vi "Display.vi"(8 "error in (no error)":errorcluster, 11 "[V] User List in":refnum<class "[V] User List.lvclass">) -> (0 "error out":errorcluster, 3 "[V] User List out":refnum<class "[V] User List.lvclass">)   [LabVIEW 2020, in "[V] User List.lvlib" / "[V] User List.lvclass"]
uses:
  [V] User List.lvclass
  [V] User List.lvclass/[V] User List.ctl
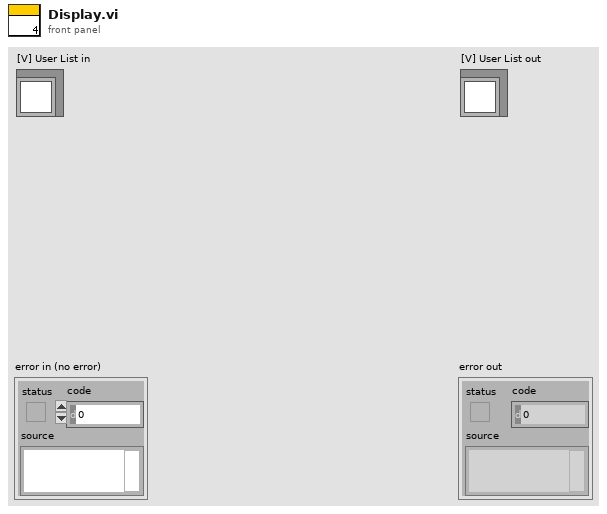
[diagram p1: front panel]
types:
  T1 = typedef "[V] User List.lvlib/[V] User List.lvclass/User Info List.ctl" = cluster{"username":string, "authority":string, "department":string, "post":string, "remark":string, "create time":timestamp, "last login time":timestamp}[]
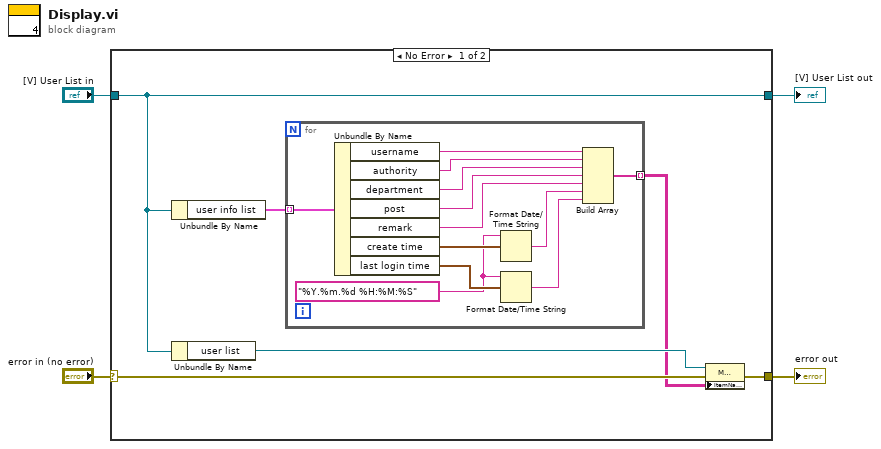
[diagram p0: block diagram]
diagram:
  n1 = case shown="No Error" "error in (no error)" {
    selector: "error in (no error)" -> [w8 w24]
    tunnel: [w5 w24] -> w3
    tunnel: [w9 w23] -> w1
    tunnel: "[V] User List in" -> [w9 w23]
    frame No Error {
      n2 = Unbundle By Name(w9) -> ("user info list"=w10:T1)
      n3 = Unbundle By Name(w9) -> ("user list"=w7:refnum<vi>)
      n4 = for {
        tunnel: w10 -> [w22] mode=indexing
        tunnel: [w16] -> w6 mode=indexing
        w11 = "%Y.%m.%d %H:%M:%S" ("time format string (%c)")
        n5 = Unbundle By Name(w22) -> ("username"=w21:string, "authority"=w17:string, "department"=w20:string, "post"=w19:string, "remark"=w18:string, "create time"=w15:timestamp, "last login time"=w14:timestamp)
        n6 = Format Date/Time String(time format string (%c)=w11, seconds (now)=w15) -> (date/time string=w13:string)  [unwired: 1 in]
        n7 = Format Date/Time String(time format string (%c)=w11, seconds (now)=w14) -> (date/time string=w12:string)  [unwired: 1 in]
        n8 = Build Array(w21, w17, w20, w19, w18, w13, w12) -> (w16:string[])
      }
      n9 = property class="MCListbox (strict)"(reference=w7, error in=w8, "ItemNames"=w6) -> (error out=w5:errorcluster)  [unwired: 1 out]
    }
    frame Error {
    }
  }
  "error out" <- w3
  "[V] User List out" <- w1
